vi "navX Example v2.vi"() -> ()   [LabVIEW 2014]
uses:
  navX Library v2/TypeDefs/Flags/Z900_navX_Flags_HardwareRevTypeDef.ctl
  navX Library v2/TypeDefs/Flags/Z900_navX_Flags_OmnimountConfigTypeDef.ctl
  navX Library v2/TypeDefs/Flags/Z900_navX_Flags_OpStatusTypeDef.ctl
  navX Library v2/TypeDefs/Flags/Z900_navX_Flags_CalibrationStatusTypeDef.ctl
  navX Library v2/TypeDefs/Flags/Z900_navX_Flags_SelfTestStatusTypeDef.ctl
  navX Library v2/TypeDefs/Z900_navX_SerialStreamTypeDef.ctl
  NI WPI/WPI_SerialPort_USB.ctl
  <vilib>/Rock Robotics/SystemInterfaces/i2clib/i2c_bus.ctl
  <vilib>/Rock Robotics/SystemInterfaces/spilib/spi_bus.ctl
  navX Library v2/IO/Open/Z900_navX_Open_Serial.vi
  navX Library v2/IO/Open/Z900_navX_Open_I2C.vi
  navX Library v2/IO/Open/Z900_navX_Open_SPI.vi
  navX Library v2/navX Library v2.lvlib
  NI WPI/NI WPI Serial USB.lvlib
panel:
  out "Connected":bool
  out "ERROR!":bool
  in  "Enable Logs":bool
  in  "Clear Log":bool
  out "Internal Error Log":errorcluster[](array[cluster])
  out "Log Size":i32
  in  "Interface Control":enum32{"Serial", "I2C", "SPI"}(tab)
  in  "Serial Port":T1=enum."MXP TTL"
  in  "Update Stream Type":bool
  in  "Stream Type":T2=enum."AHRS"
  in  "I2C Bus":T3=enum."I2C MXP"
  in  "SPI Bus":T4=enum."SPI MXP"
  in  "Zero Yaw":bool
  out "Raw Values":T5
  out "Quaternion":T6
  out "Linear Acceleration":T7
  out "Displacement":T8
  out "Offsets":T9
  out "Timestamp":u32
  out "MPUTemp":dbl(slide) scale=20.0..50.0
  in  "Update Rate":u8=50 min=4 max=50
  out "Status":T13 {"OP Status" items=["INITIALIZING", "SELFTEST_IN_PROGRESS", "ERROR", "IMU_AUTOCAL_IN_PROGRESS", "NORMAL"]; "Calibration Status" items=["IMU_CAL_STATE_MASK"=3, "IMU_CAL_STATE_INPROGRESS"=0, "IMU_CAL_STATE_ACCUMULATE"=1, "IMU_CAL_STATE_COMPLETE"=2]; "Self Test Status" items=["STATUS_COMPLETE"=128, "RESULT_GYRO_PASSED"=1, "RESULT_ACCEL_PASSED"=2, "RESULT_MAG_PASSED"=4, "RESULT_BARO_PASSED"=8]}
  out "Board Information":T16 {"Board"."Hardware Revision" items=["navX-MXP"=33, "navX-Micro"=40]; "Omnimount Config" items=["DEFAULT", "X_UP", "X_DOWN", "Y_UP", "Y_DOWN", "Z_UP", "Z_DOWN"]}
  out "YRPHfH":T17
  in  "stop":bool
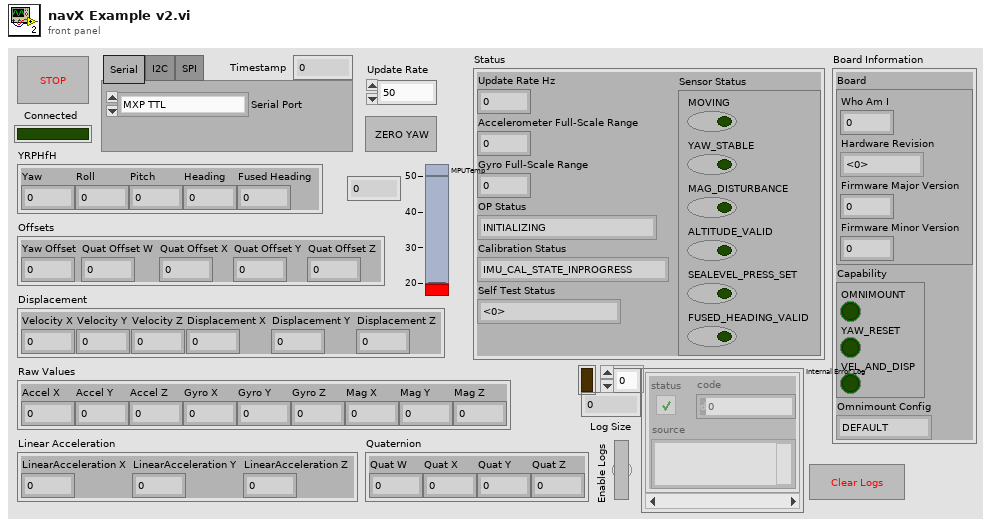
[diagram p1: front panel]
types:
  T1 = typedef "NI WPI Serial USB.lvlib/WPI_SerialPort_USB.ctl" = enum16{"Onboard RS-232", "MXP TTL", "USB"}
  T2 = typedef "navX Library v2.lvlib/Z900_navX_SerialStreamTypeDef.ctl" = enum16{"YRPH", "Quadernion", "Gyro/Raw", "AHRS", "AHRSAndPositioning"}
  T3 = typedef "i2c_bus.ctl" = enum16{"I2C On-Board", "I2C MXP", "Invalid"}
  T4 = typedef "spi_bus.ctl" = enum16{"SPI On-Board, CS0", "SPI On-Board, CS1", "SPI On-Board, CS2", "SPI On-Board, CS3", "SPI MXP", "Invalid"}
  T5 = cluster{"Accel X":dbl, "Accel Y":dbl, "Accel Z":dbl, "Gyro X":dbl, "Gyro Y":dbl, "Gyro Z":dbl, "Mag X":dbl, "Mag Y":dbl, "Mag Z":dbl}
  T6 = cluster{"Quat W":dbl, "Quat X":dbl, "Quat Y":dbl, "Quat Z":dbl}
  T7 = cluster{"LinearAcceleration X":dbl, "LinearAcceleration Y":dbl, "LinearAcceleration Z":dbl}
  T8 = cluster{"Velocity X":dbl, "Velocity Y":dbl, "Velocity Z":dbl, "Displacement X":dbl, "Displacement Y":dbl, "Displacement Z":dbl}
  T9 = cluster{"Yaw Offset":dbl, "Quat Offset W":dbl, "Quat Offset X":dbl, "Quat Offset Y":dbl, "Quat Offset Z":dbl}
  T10 = typedef "navX Library v2.lvlib/Z900_navX_Flags_OpStatusTypeDef.ctl" = u8
  T11 = typedef "navX Library v2.lvlib/Z900_navX_Flags_CalibrationStatusTypeDef.ctl" = u8
  T12 = typedef "navX Library v2.lvlib/Z900_navX_Flags_SelfTestStatusTypeDef.ctl" = u8
  T13 = cluster{"Update Rate Hz":u8, "Accelerometer Full-Scale Range":u8, "Gyro Full-Scale Range":u16, "OP Status":T10, "Calibration Status":T11, "Self Test Status":T12, "Sensor Status":cluster{"MOVING":bool, "YAW_STABLE":bool, "MAG_DISTURBANCE":bool, "ALTITUDE_VALID":bool, "SEALEVEL_PRESS_SET":bool, "FUSED_HEADING_VALID":bool}}
  T14 = typedef "navX Library v2.lvlib/Z900_navX_Flags_HardwareRevTypeDef.ctl" = u8
  T15 = typedef "navX Library v2.lvlib/Z900_navX_Flags_OmnimountConfigTypeDef.ctl" = u8
  T16 = cluster{"Board":cluster{"Who Am I":u8, "Hardware Revision":T14, "Firmware Major Version":u8, "Firmware Minor Version":u8}, "Capability":cluster{"OMNIMOUNT":bool, "YAW_RESET":bool, "VEL_AND_DISP":bool}, "Omnimount Config":T15}
  T17 = cluster{"Yaw":dbl, "Roll":dbl, "Pitch":dbl, "Heading":dbl, "Fused Heading":dbl}
  T18 = cluster{"Interface Control":enum32{"Serial", "I2C", "SPI"}, "Serial Port":T1, "I2C Bus":T3, "SPI Bus":T4, u8}
  T19 = cluster{"Interface Control":bool, "Serial Port":bool, "I2C Bus":bool, "SPI Bus":bool, bool}
  T20 = typedef "navX Library v2.lvlib/Z900_navX_DeviceTypeDef.ctl" = cluster{"Interface":cluster{"Protocol":T21, "Update Rate (4Hz-60Hz)":u8, "navX Open TypeDef":variant}, "Notify Packet":refnum<notifier>, "Loop VI Refnum":refnum<vi>, "Ready to Close Occurrence Refnum":refnum<k4>}
  T21 = typedef "navX Library v2.lvlib/Z900_navX_ProtocolTypeDef.ctl" = enum16{"SERIAL", "I2C", "SPI"}
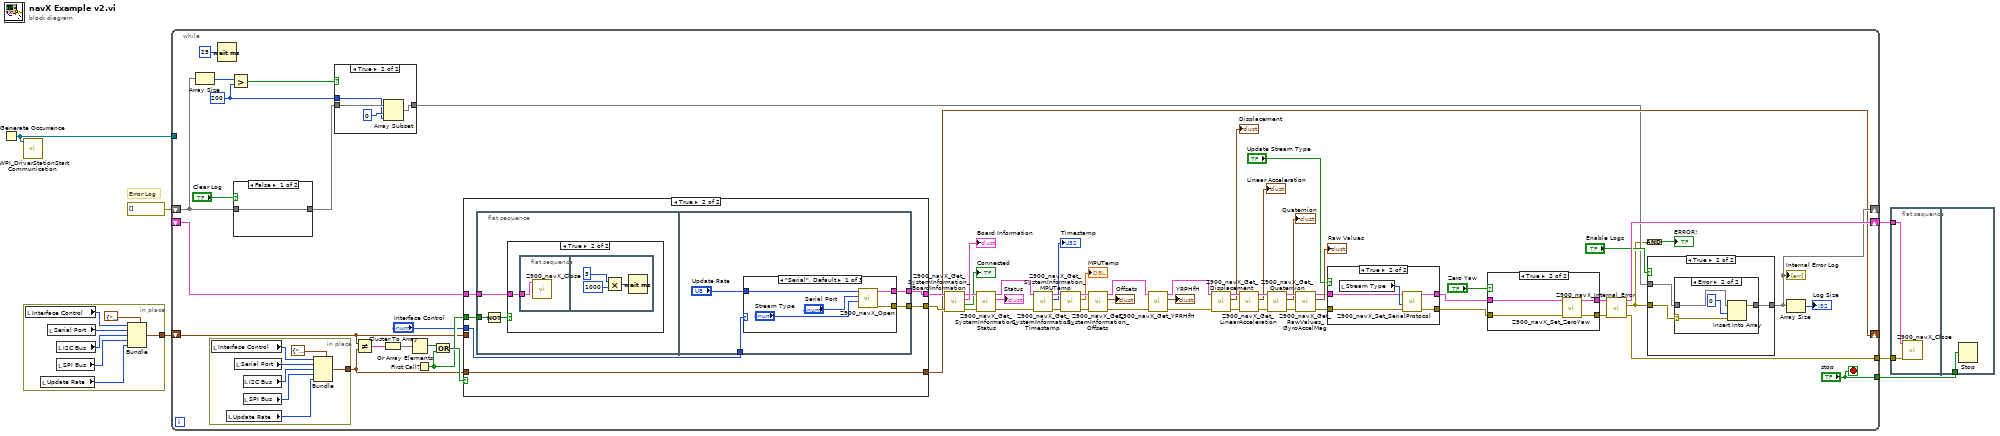
[diagram p0: block diagram]
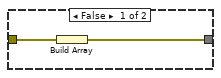
[diagram p3: hidden frame]
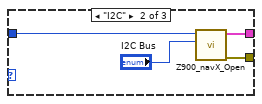
[diagram p7: hidden frame]
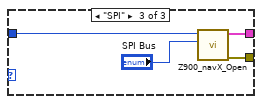
[diagram p8: hidden frame]
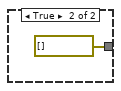
[diagram p9: hidden frame]
diagram:
  # "Error Log"
  n1 = Generate Occurrence() -> (w2:refnum<k4>)
  n2 = call <vilib>:"WPI_DriverStationStart Communication.vi"("occurrence"=w2) -> ()  [unwired: 11 in]
  n3 = in-place {
    in-place-border: [w12] -> w3
    n4 = local read "Interface Control"() -> (w11:enum32{"Serial", "I2C", "SPI"})
    n5 = local read "Update Rate"() -> (w7:u8)
    n6 = local read "Serial Port"() -> (w10:T1)
    n7 = local read "I2C Bus"() -> (w9:T3)
    n8 = local read "SPI Bus"() -> (w8:T4)
    n9 = Bundle(cluster=T18 {"Interface Control"=enum."Serial", "Serial Port"=enum."Onboard RS-232", "I2C Bus"=enum."I2C On-Board", "SPI Bus"=enum."SPI On-Board, CS0", 0} ("output cluster"), "Interface Control"=w11, "Serial Port"=w10, "I2C Bus"=w9, "SPI Bus"=w8, w7) -> (w12:T18)
  }
  n10 = while {
    shift-right: [w41] -> w6
    shift-left: _ -> [w38]
    shift-right: [w40] -> _
    shift-left: errorcluster[] [] -> [w23]
    tunnel: [w35] -> w4
    shift-right: [w28] -> _
    shift-left: w3 -> [w27]
    tunnel: w2 -> [_]
    tunnel: ["stop"] -> w1
    stop <- "stop" stop-if-true
    w17 = 200 ("y")
    n11 = Array Size(array=w23) -> (size(s)=w22:i32)
    n12 = in-place {
      in-place-border: [w89] -> w24
      n13 = local read "Interface Control"() -> (w88:enum32{"Serial", "I2C", "SPI"})
      n14 = local read "Update Rate"() -> (w84:u8)
      n15 = local read "Serial Port"() -> (w87:T1)
      n16 = local read "I2C Bus"() -> (w86:T3)
      n17 = local read "SPI Bus"() -> (w85:T4)
      n18 = Bundle(cluster=T18 {"Interface Control"=enum."Serial", "Serial Port"=enum."Onboard RS-232", "I2C Bus"=enum."I2C On-Board", "SPI Bus"=enum."SPI On-Board, CS0", 0} ("output cluster"), "Interface Control"=w88, "Serial Port"=w87, "I2C Bus"=w86, "SPI Bus"=w85, w84) -> (w89:T18)
    }
    n19 = Wait (ms)(milliseconds to wait=u32 25) -> ()  [unwired: 1 out]
    n20 = Greater?(x=w22, y=w17) -> (0:w20:bool)
    n21 = case shown="False" "Clear Log" {
      tunnel: [w134 errorcluster[] []] -> w19
      tunnel: w23 -> [w134 _]
      frame False {
      }
      frame True {
      }
    }
    n22 = case shown="True" w20 {
      tunnel: [w79 w80] -> w18
      tunnel: w19 -> [w79 w83]
      tunnel: w17 -> [_ w81]
      frame False {
      }
      frame True {
        n23 = Array Subset(array=w83, index=0, length=w81) -> (w80:errorcluster[])
      }
    }
    n24 = Not Equal?(x=w27, y=w24) -> (x != y?=w31:T19)
    n25 = Cluster To Array(cluster=w31) -> (array=w30:bool[])
    n26 = Or Array Elements(Boolean array=w30) -> (logical OR=w29:bool)
    n27 = First Call?() -> (First Call?: T/F=w33:bool)
    n28 = Or(x=w29, y=w33) -> (x .or. y?=w34:bool)
    n29 = case shown="True" w34 {
      tunnel: w38 -> [w102 w108]
      tunnel: [w102 w107] -> w37
      tunnel: [_ w106] -> w36
      tunnel: "Interface Control" -> [_ w105]
      tunnel: w33 -> [_ w104]
      tunnel: w24 -> [_ w103]
      tunnel: [w101 w103] -> w28
      tunnel: w27 -> [w101 _]
      frame False {
      }
      frame True {
        n30 = flat-sequence {
          tunnel: w104 -> [w109]
          tunnel: w108 -> [w110]
          tunnel: [w119] -> w107
          tunnel: [w118] -> w106
          tunnel: w105 -> [w117]
          frame #0 {
            n31 = Not(x=w109) -> (.not. x?=w111:bool)
            n32 = case shown="True" w111 {
              tunnel: w110 -> [_ w112]
              frame False {
              }
              frame True {
                n33 = flat-sequence {
                  tunnel: w112 -> [w113]
                  frame #0 {
                    n34 = call "Z900_navX_Close.vi"("navX Device"=w113) -> ()  [unwired: 10 in, 1 out]
                  }
                  frame #1 {
                    n35 = Multiply(x=u32 3, y=u32 1000 ("x")) -> (x*y=w115:u32)
                    n36 = Wait (ms)(milliseconds to wait=w115) -> ()  [unwired: 1 out]
                  }
                }
              }
            }
          }
          frame #1 {
            n37 = case shown="\"Serial\", Default" w117 {
              tunnel: [w123 w127 w132] -> w119
              tunnel: [w122 w126 w131] -> w118
              tunnel: "Update Rate" -> [w121 w129 w130]
              frame "Serial", Default {
                n38 = call-poly "Z900_navX_Open.vi"("Stream Type"="Stream Type", "Serial Port"="Serial Port", "Update Rate (4Hz-60Hz)"=w121) -> ("error out"=w122:errorcluster, "navX Device"=w123:T20)  [unwired: 7 in]
              }
              frame "I2C" {
                n39 = call-poly "Z900_navX_Open.vi"("I2C Bus"="I2C Bus", "Update Rate (4Hz-60Hz)"=w129) -> ("error out"=w126:errorcluster, "navX Device"=w127:T20)  [unwired: 8 in]
              }
              frame "SPI" {
                n40 = call-poly "Z900_navX_Open.vi"("SPI Bus"="SPI Bus", "Update Rate (4Hz-60Hz)"=w130) -> ("error out"=w131:errorcluster, "navX Device"=w132:T20)  [unwired: 8 in]
              }
            }
          }
        }
      }
    }
    n41 = call "Z900_navX_Get_SystemInformation_BoardInformation.vi"("error in (no error)"=w36, "navX Device"=w37) -> ("error out"=w75:errorcluster, "Connected"=→"Connected":bool, "Board Information"=→"Board Information":T16, "navX Device"=w74:T20)  [unwired: 6 in]
    n42 = call "Z900_navX_Get_SystemInformation_Status.vi"("error in (no error)"=w75, "navX Device"=w74) -> ("error out"=w72:errorcluster, "Status"=→"Status":T13, "navX Device"=w71:T20)  [unwired: 6 in, 1 out]
    n43 = call "Z900_navX_Get_SystemInformation_Timestamp.vi"("error in (no error)"=w72, "navX Device"=w71) -> ("error out"=w69:errorcluster, "Timestamp"=→"Timestamp":u32, "navX Device"=w70:T20)  [unwired: 6 in, 1 out]
    n44 = call "Z900_navX_Get_SystemInformation_MPUTemp.vi"("error in (no error)"=w69, "navX Device"=w70) -> ("error out"=w67:errorcluster, "MPUTemp"=→"MPUTemp":dbl, "navX Device"=w68:T20)  [unwired: 6 in, 1 out]
    n45 = call "Z900_navX_Get_SystemInformation_Offsets.vi"("error in (no error)"=w67, "navX Device"=w68) -> ("error out"=w65:errorcluster, "Offsets"=→"Offsets":T9, "navX Device"=w66:T20)  [unwired: 6 in, 1 out]
    n46 = call "Z900_navX_Get_YPRHfH.vi"("error in (no error)"=w65, "navX Device"=w66) -> ("error out"=w63:errorcluster, "YRPHfH"=→"YRPHfH":T17, "navX Device"=w64:T20)  [unwired: 6 in, 1 out]
    n47 = call "Z900_navX_Get_Displacement.vi"("error in (no error)"=w63, "navX Device"=w64) -> ("error out"=w61:errorcluster, "Displacement"=→"Displacement":T8, "navX Device"=w62:T20)  [unwired: 6 in, 1 out]
    n48 = call "Z900_navX_Get_LinearAcceleration.vi"("error in (no error)"=w61, "navX Device"=w62) -> ("error out"=w59:errorcluster, "Linear Acceleration"=→"Linear Acceleration":T7, "navX Device"=w60:T20)  [unwired: 6 in, 1 out]
    n49 = call "Z900_navX_Get_Quaternion.vi"("error in (no error)"=w59, "navX Device"=w60) -> ("error out"=w57:errorcluster, "Quaternion"=→"Quaternion":T6, "navX Device"=w58:T20)  [unwired: 6 in, 1 out]
    n50 = call "Z900_navX_Get_RawValues_GyroAccelMag.vi"("error in (no error)"=w57, "navX Device"=w58) -> ("error out"=w47:errorcluster, "Raw Values"=→"Raw Values":T5, "navX Device"=w48:T20)  [unwired: 6 in, 1 out]
    n51 = case shown="True" "Update Stream Type" {
      tunnel: w48 -> [w143 w147]
      tunnel: [w143 w146] -> w46
      tunnel: w47 -> [w142 w145]
      tunnel: [w142 w144] -> w45
      frame False {
      }
      frame True {
        n52 = local read "Stream Type"() -> (w148:T2)
        n53 = call "Z900_navX_Set_SerialProtocol.vi"("error in (no error)"=w145, "Stream Type"=w148, "navX Device"=w147) -> ("error out"=w144:errorcluster, "navX Device"=w146:T20)  [unwired: 7 in]
      }
    }
    n54 = case shown="True" "Zero Yaw" {
      tunnel: w46 -> [w137 w141]
      tunnel: [w137 w140] -> w43
      tunnel: w45 -> [w136 w139]
      tunnel: [w136 w138] -> w42
      frame False {
      }
      frame True {
        n55 = call "Z900_navX_Set_ZeroYaw.vi"("error in (no error)"=w139, "navX Device"=w141) -> ("error out"=w138:errorcluster, "navX Device"=w140:T20)  [unwired: 8 in]
      }
    }
    n56 = call "Z900_navX_Internal_Error.vi"("error in (no error)"=w42, "navX Device"=w43) -> ("error out"=w35:errorcluster, "Internal error out"=w16:errorcluster, "navX Device"=w41:T20)  [unwired: 7 in]
    n57 = Compound Arithmetic op=AND(w16) -> (→"ERROR!":bool)
    n58 = case shown="True" "Enable Logs" {
      tunnel: w16 -> [w92 w95]
      tunnel: [w91 w94] -> w40
      tunnel: w18 -> [_ w93]
      frame False {
        n59 = Build Array(w92) -> (w91:errorcluster[])
      }
      frame True {
        n60 = case shown="Error" w95 {
          selector: w95 -> [_ w99]
          tunnel: [w96 w97] -> w94
          tunnel: w93 -> [w96 w100]
          frame No Error {
          }
          frame Error {
            n61 = Insert Into Array(array=w100, index=0, new element=w99) -> (w97:errorcluster[])
          }
        }
      }
    }
    "Internal Error Log" <- w40
    n62 = Array Size(array=w40) -> (size(s)=→"Log Size":i32)
  }
  n63 = flat-sequence {
    tunnel: w6 -> [w150]
    tunnel: w4 -> [w149]
    tunnel: w1 -> [w151]
    frame #0 {
      n64 = call "Z900_navX_Close.vi"("error in (no error)"=w149, "navX Device"=w150) -> ()  [unwired: 9 in, 1 out]
    }
    frame #1 {
      n65 = Stop(stop? (T)=w151) -> ()
    }
  }
